vi "Create_filter_points_Sub.vi"(1 "Numeric Value?":bool[](array[boolean]), 4 "No of filter options":i32=100, 5 "Precision":string, 6 "Tolerance":dbl=1.0 format="%.2f", 7 "Bin Matches in":bool[][](array[boolean]), 8 "Numeric Array":dbl[](array[numeric]) format="%.2f", 9 "Bin Names In":string[](array[string]), 10 "String Array":string[](array[string])) -> (2 "Bin Matches":bool[][](array[boolean]), 3 "Bin Names":string[](array[string]))   [LabVIEW 2010]
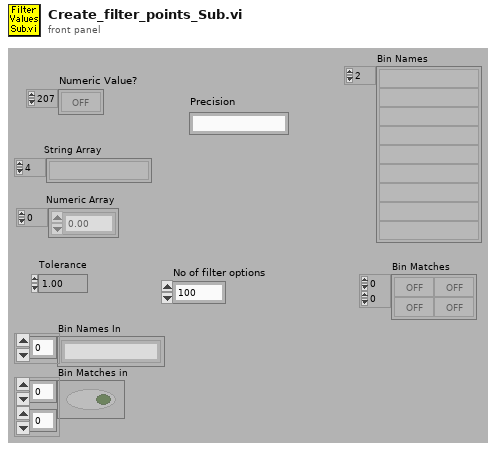
[diagram p1: front panel]
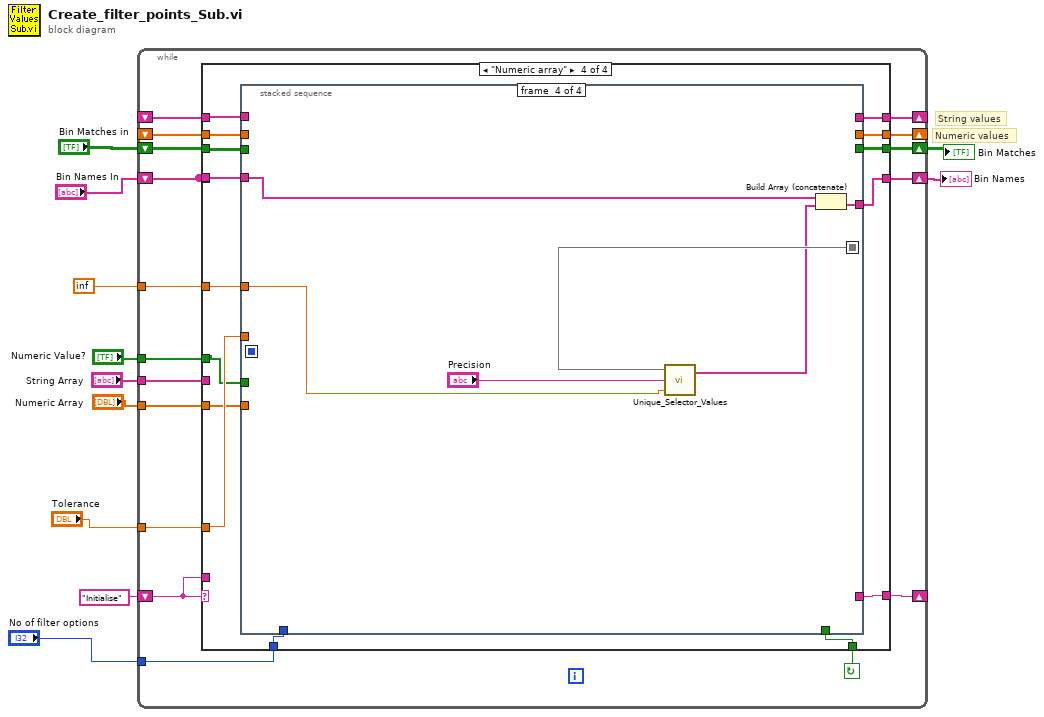
[diagram p0: block diagram]
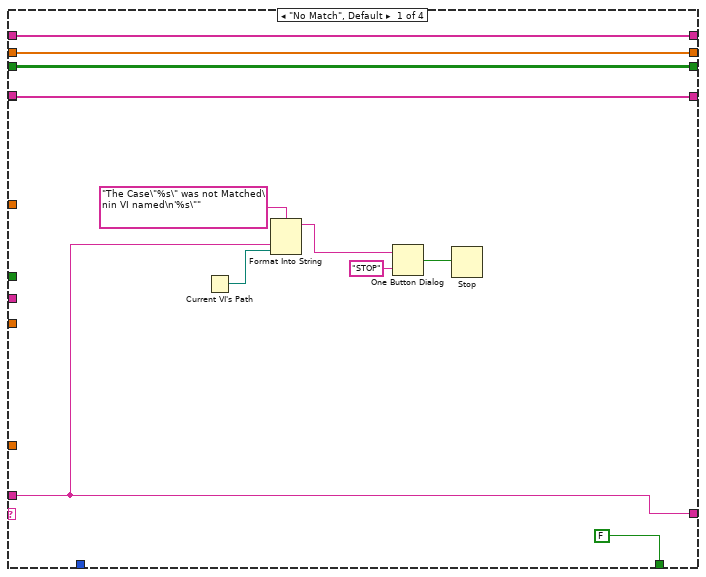
[diagram p2: hidden frame]
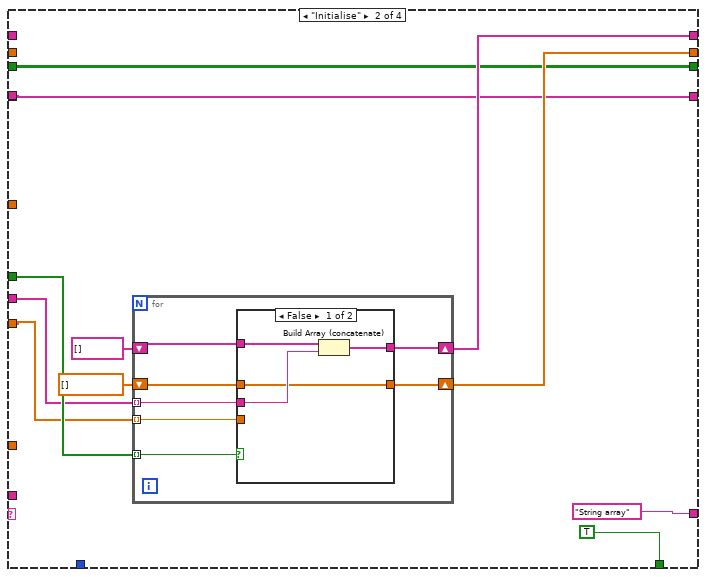
[diagram p3: hidden frame]
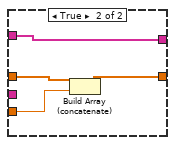
[diagram p4: hidden frame]
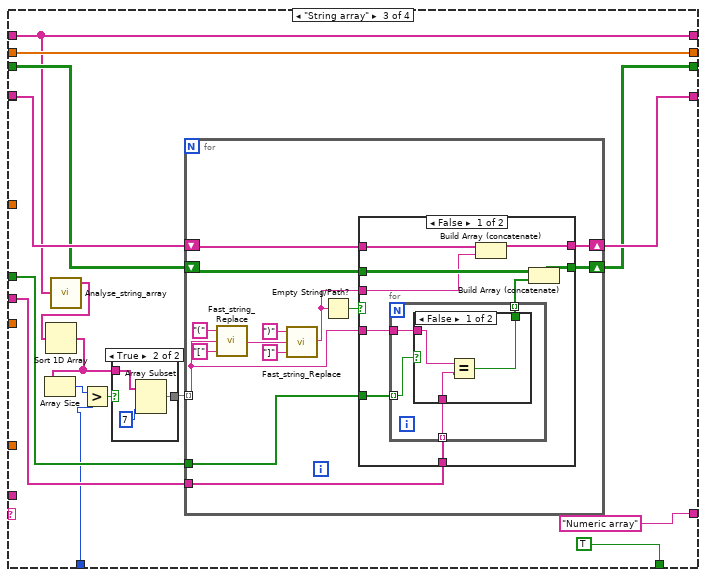
[diagram p5: hidden frame]
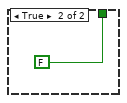
[diagram p7: hidden frame]
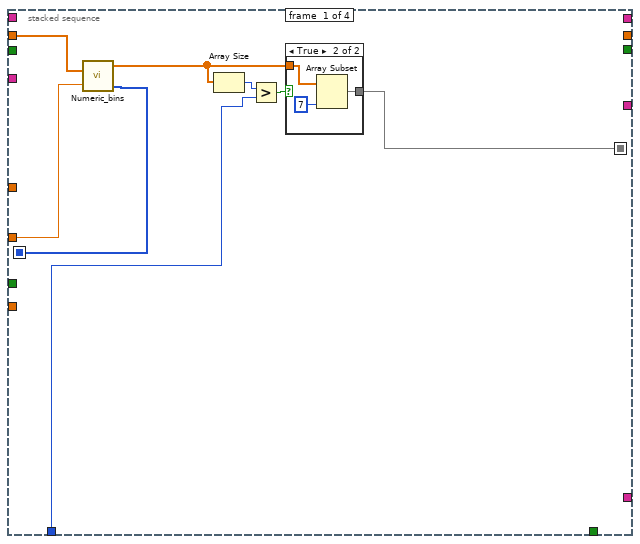
[diagram p9: hidden frame]
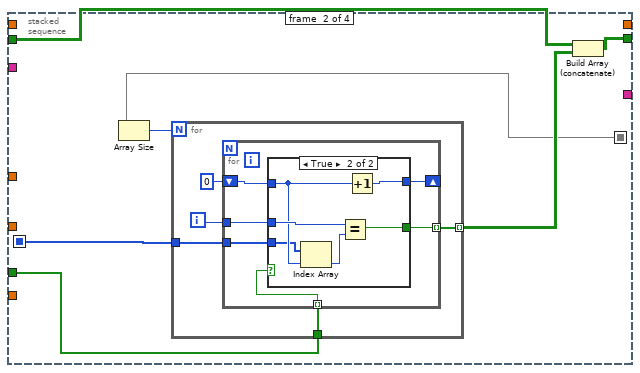
[diagram p11: hidden frame]
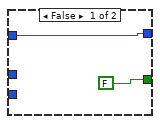
[diagram p12: hidden frame]
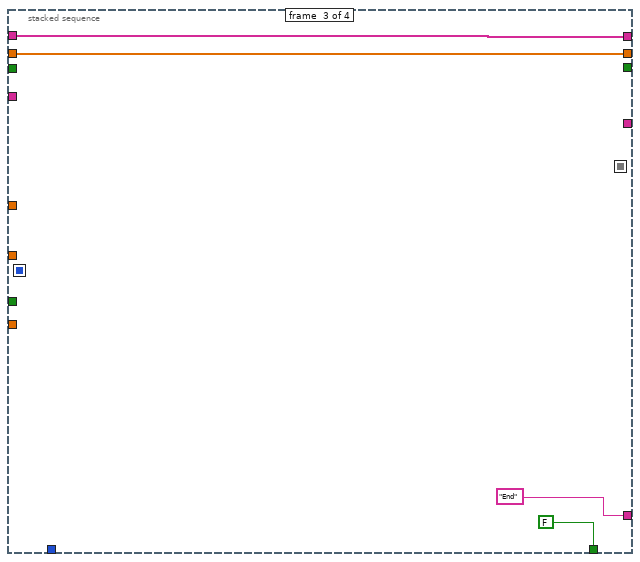
[diagram p13: hidden frame]
diagram:
  # "String values"
  # "Numeric values"
  n1 = while {
    tunnel: "Numeric Value?" -> [w15]
    shift-left: _ -> [w17]
    shift-right: [w16] -> _
    shift-left: "Bin Names In" -> [w18]
    shift-right: [w19] -> w10
    tunnel: "Tolerance" -> [w20]
    shift-left: "Bin Matches in" -> [w24]
    shift-right: [w23] -> w8
    shift-left: _ -> [w21]
    shift-right: [w27] -> _
    shift-left: "Initialise" -> [w22]
    shift-right: [w26] -> _
    tunnel: inf -> [w28]
    tunnel: "Numeric Array" -> [w14]
    tunnel: "String Array" -> [w13]
    tunnel: "No of filter options" -> [w12]
    stop <- w25 continue-if-true
    n2 = case shown="\"Numeric array\"" w22 {
      tunnel: w28 -> [_ _ _ w125]
      tunnel: [w38 w42 w80 w129] -> w27
      tunnel: [w29 "String array" "Numeric array" w132] -> w26
      tunnel: [FALSE TRUE TRUE w133] -> w25
      tunnel: w24 -> [w37 w40 w76 w127]
      tunnel: [w37 w40 w75 w126] -> w23
      tunnel: w22 -> [w29 _ _ _]
      tunnel: w21 -> [w38 _ w80 w128]
      tunnel: w20 -> [_ _ _ w130]
      tunnel: [w36 w41 w77 w131] -> w19
      tunnel: w18 -> [w36 w41 w78 w122]
      tunnel: w18 -> [_ _ _ _]
      tunnel: w17 -> [w35 _ w74 w124]
      tunnel: [w35 w43 w74 w123] -> w16
      tunnel: w15 -> [_ w48 w72 w121]
      tunnel: w14 -> [_ w45 _ w120]
      tunnel: w13 -> [_ w47 w73 _]
      tunnel: w12 -> [_ _ w66 w119]
      frame "No Match", Default {
        n3 = Current VI's Path() -> (path=w30:path)
        n4 = Format Into String(format string="The Case\"%s\" was not Matched\nin VI named\n'%s\"" ("Format String"), w29, w30) -> (resulting string=w33:string)  [unwired: 2 in, 1 out]
        n5 = One Button Dialog(message=w33, button name ("OK")="STOP") -> (true=w31:bool)
        n6 = Stop(stop? (T)=w31) -> ()
      }
      frame "Initialise" {
        n7 = for {
          tunnel: w48 -> [w57] mode=indexing
          shift-right: [w55] -> w43
          shift-left: string[] [] -> [w56]
          shift-right: [w52] -> w42
          shift-left: dbl[] [] -> [w53]
          tunnel: w47 -> [w54] mode=indexing
          tunnel: w45 -> [w51] mode=indexing
          n8 = case shown="False" w57 {
            tunnel: w56 -> [w61 w62]
            tunnel: [w60 w62] -> w55
            tunnel: w54 -> [w59 _]
            tunnel: w53 -> [w58 w65]
            tunnel: [w58 w64] -> w52
            tunnel: w51 -> [_ w63]
            frame False {
              n9 = Build Array (concatenate)(w61, w59) -> (w60:string[])
            }
            frame True {
              n10 = Build Array (concatenate)(w65, w63) -> (w64:dbl[])
            }
          }
        }
      }
      frame "String array" {
        n11 = call "Analyse_string_array.vi"("String array"=w74) -> ("Unique strings"=w71:string[])  [unwired: 2 out]
        n12 = Sort 1D Array(array=w71) -> (sorted array=w68:string[])
        n13 = Array Size(array=w68) -> (size(s)=w69:i32)
        n14 = Greater?(x=w69, y=w66) -> (0:w70:bool)
        n15 = case shown="True" w70 {
          tunnel: w68 -> [w82 w85]
          tunnel: [w82 w84] -> w67
          frame False {
          }
          frame True {
            n16 = Array Subset(array=w85, length=7) -> (w84:string[])  [unwired: 1 in]
          }
        }
        n17 = for {
          tunnel: w73 -> [w89]
          tunnel: w67 -> [w88] mode=indexing
          shift-right: [w92] -> w77
          shift-left: w78 -> [w93]
          shift-right: [w90] -> w75
          shift-left: w76 -> [w91]
          tunnel: w72 -> [w86]
          n18 = call "Fast_string_Replace.vi"("Replace match with:"="[", "Input String"=w88, "regular expression"="(") -> ("Output String"=w95:string)  [unwired: 2 out]
          n19 = call "Fast_string_Replace.vi"("Replace match with:"="]", "Input String"=w95, "regular expression"=")") -> ("Output String"=w87:string)  [unwired: 2 out]
          n20 = Empty String/Path?(string/path=w87) -> (empty?=w94:bool)
          n21 = case shown="False" w94 {
            tunnel: w93 -> [w108 w118]
            tunnel: [w107 w118] -> w92
            tunnel: w91 -> [w106 w117]
            tunnel: [w105 w117] -> w90
            tunnel: w88 -> [w104 _]
            tunnel: w89 -> [w103 _]
            tunnel: w87 -> [w101 _]
            tunnel: w86 -> [w100 _]
            frame False {
              n22 = for {
                tunnel: w104 -> [w112]
                tunnel: w103 -> [w111] mode=indexing
                tunnel: [w110] -> w102 mode=indexing
                tunnel: w100 -> [w109] mode=indexing
                n23 = case shown="False" w109 {
                  tunnel: w112 -> [w115 _]
                  tunnel: w111 -> [w114 _]
                  tunnel: [w113 FALSE] -> w110
                  frame False {
                    n24 = Equal?(x=w115, y=w114) -> (x = y?=w113:bool)
                  }
                  frame True {
                  }
                }
              }
              n25 = Build Array (concatenate)(w108, w101) -> (w107:string[])
              n26 = Build Array (concatenate)(w106, w102) -> (w105:bool[][])
            }
            frame True {
            }
          }
        }
      }
      frame "Numeric array" {
        n27 = stacked-sequence {
          seq-local: [w134 _ _ _] -> [_ w147 _ w179]
          seq-local: [w139 _ _ _] -> [_ w150 _ _]
          tunnel: w130 -> [w140 _ _ _]
          tunnel: [_ _ w172 _] -> w129
          tunnel: w128 -> [w141 _ w172 _]
          tunnel: w127 -> [_ w152 _ _]
          tunnel: [_ w151 _ _] -> w126
          tunnel: [_ _ FALSE _] -> w133
          tunnel: [_ _ "End" _] -> w132
          tunnel: w125 -> [_ _ _ w176]
          tunnel: [_ _ _ w181] -> w131
          tunnel: w124 -> [_ _ w173 _]
          tunnel: [_ _ w173 _] -> w123
          tunnel: w122 -> [_ _ _ w180]
          tunnel: w121 -> [_ w149 _ _]
          tunnel: w120 -> [_ _ _ _]
          tunnel: w119 -> [w136 _ _ _]
          frame #0 {
            n28 = call "Numeric_bins.vi"("Values"=w141, "Tolerance"=w140) -> ("Bin Centres"=w135:dbl[], "Bin Index"=w139:i32[])  [unwired: 1 out]
            n29 = Array Size(array=w135) -> (size(s)=w138:i32)
            n30 = Greater?(x=w138, y=w136) -> (0:w137:bool)
            n31 = case shown="True" w137 {
              tunnel: w135 -> [w142 w145]
              tunnel: [w142 w144] -> w134
              frame False {
              }
              frame True {
                n32 = Array Subset(array=w145, length=7) -> (w144:dbl[])  [unwired: 1 in]
              }
            }
          }
          frame #1 {
            n33 = Array Size(array=w147) -> (size(s)=w146:i32)
            n34 = for {
              N: w146 -> [_]
              tunnel: w150 -> [w157]
              tunnel: [w156] -> w148 mode=indexing
              tunnel: w149 -> [w155]
              i -> [w153]
              n35 = for {
                tunnel: w157 -> [w159]
                tunnel: w153 -> [w160]
                tunnel: [w158] -> w156 mode=indexing
                tunnel: w155 -> [w163] mode=indexing
                shift-right: [w161] -> _
                shift-left: 0 -> [w162]
                n36 = case shown="True" w163 {
                  tunnel: w162 -> [w165 w169]
                  tunnel: [w165 w171] -> w161
                  tunnel: w160 -> [_ w170]
                  tunnel: w159 -> [_ w168]
                  tunnel: [FALSE w166] -> w158
                  frame False {
                  }
                  frame True {
                    n37 = Index Array(array=w168, index=w169) -> (element=w167:i32)
                    n38 = Equal?(x=w170, y=w167) -> (x = y?=w166:bool)
                    n39 = Increment(x=w169) -> (x+1=w171:i32)
                  }
                }
              }
            }
            n40 = Build Array (concatenate)(w152, w148) -> (w151:bool[][])
          }
          frame #2 {
          }
          frame #3 {
            n41 = call "Unique_Selector_Values.vi"("Number that means blank"=w176, "Precision"="Precision", "Bin Centres"=w179) -> ("Bin Strings"=w177:string[])  [unwired: 1 out]
            n42 = Build Array (concatenate)(w180, w177) -> (w181:string[])
          }
        }
      }
    }
  }
  "Bin Names" <- w10
  "Bin Matches" <- w8
